vi "95-5 Filter.vi"(1 "Reset":bool, 2 "Percent":dbl, 3 "In":dbl) -> (0 "Out":dbl)   [LabVIEW 2016]
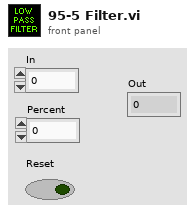
[diagram p1: front panel]
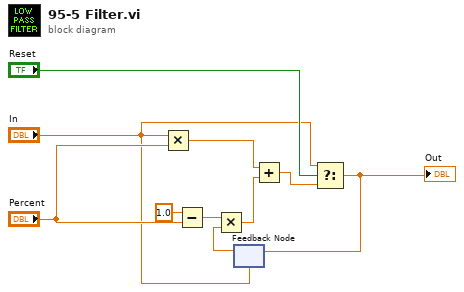
[diagram p0: block diagram]
diagram:
  n1 = Multiply(x="In", y="Percent") -> (x*y=w8:dbl)
  n2 = Subtract(x=1.0 ("y"), y="Percent") -> (x-y=w10:dbl)
  n3 = feedback #1("In") -> (w7:dbl)
  n4 = Multiply(x=w10, y=w7) -> (x*y=w9:dbl)
  n5 = Add(x=w8, y=w9) -> (x+y=w3:dbl)
  n6 = Select(t="In", s="Reset", f=w3) -> (s? t:f=w4:dbl)
  "Out" <- w4
  n7 = feedback-in #1(w4) -> ()
